vi "PrepareHWI.vi"(8 "error in (no error)":errorcluster, 9 "Master Device in":refnum<class "Master Device.lvclass">, 10 "Current Variables":T1[](array[typedef]), 11 "Slave_Pulseblaster in":refnum<class "Slave_Pulseblaster.lvclass">) -> (0 "error out":errorcluster, 2 "Master Device out":refnum<class "Master Device.lvclass">, 3 "Slave_Pulseblaster out":refnum<class "Slave_Pulseblaster.lvclass">)   [LabVIEW 2013, in "Slave_Pulseblaster.lvclass"]
doc: "Prepare HWI will parse string table values to generate a hardware image for each device. Both variables and user functions can be pre-registered! This makes setting variables optional."
uses:
  Slave_Pulseblaster.lvclass
  TypeDefs/Active procedure variables.ctl
  Master Device/Master Device.lvclass
  Slave_Pulseblaster.lvclass/Slave_Pulseblaster.ctl
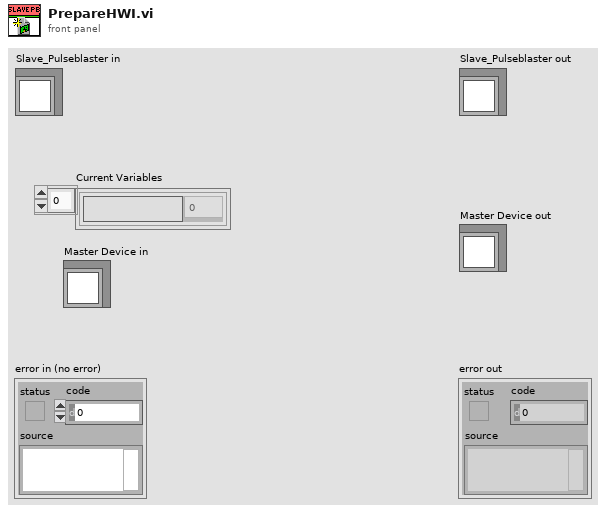
[diagram p1: front panel]
types:
  T1 = typedef "Active procedure variables.ctl" = cluster{"Procedure variable":string, "Value":dbl}
  T2 = cluster{"Output Bits":u32, "Data Field":u32, "OP Code":u8, "Delay Count":u64}[]
  T3 = cluster{"Output Bits":u32, "Data Field":u32, "OP Code":u8, "Delay Count":u64}
  T4 = typedef "SlaveInfo.ctl" = cluster{"Triggering":bool[][], "Ramp Info":T5[], "Line Inversion":bool[]}
  T5 = typedef "RampInfo.ctl" = cluster{"Table Ramp Index":i32, "Ramp Time":dbl, "Number of Steps":i32, "Instruction Array Index":i32}
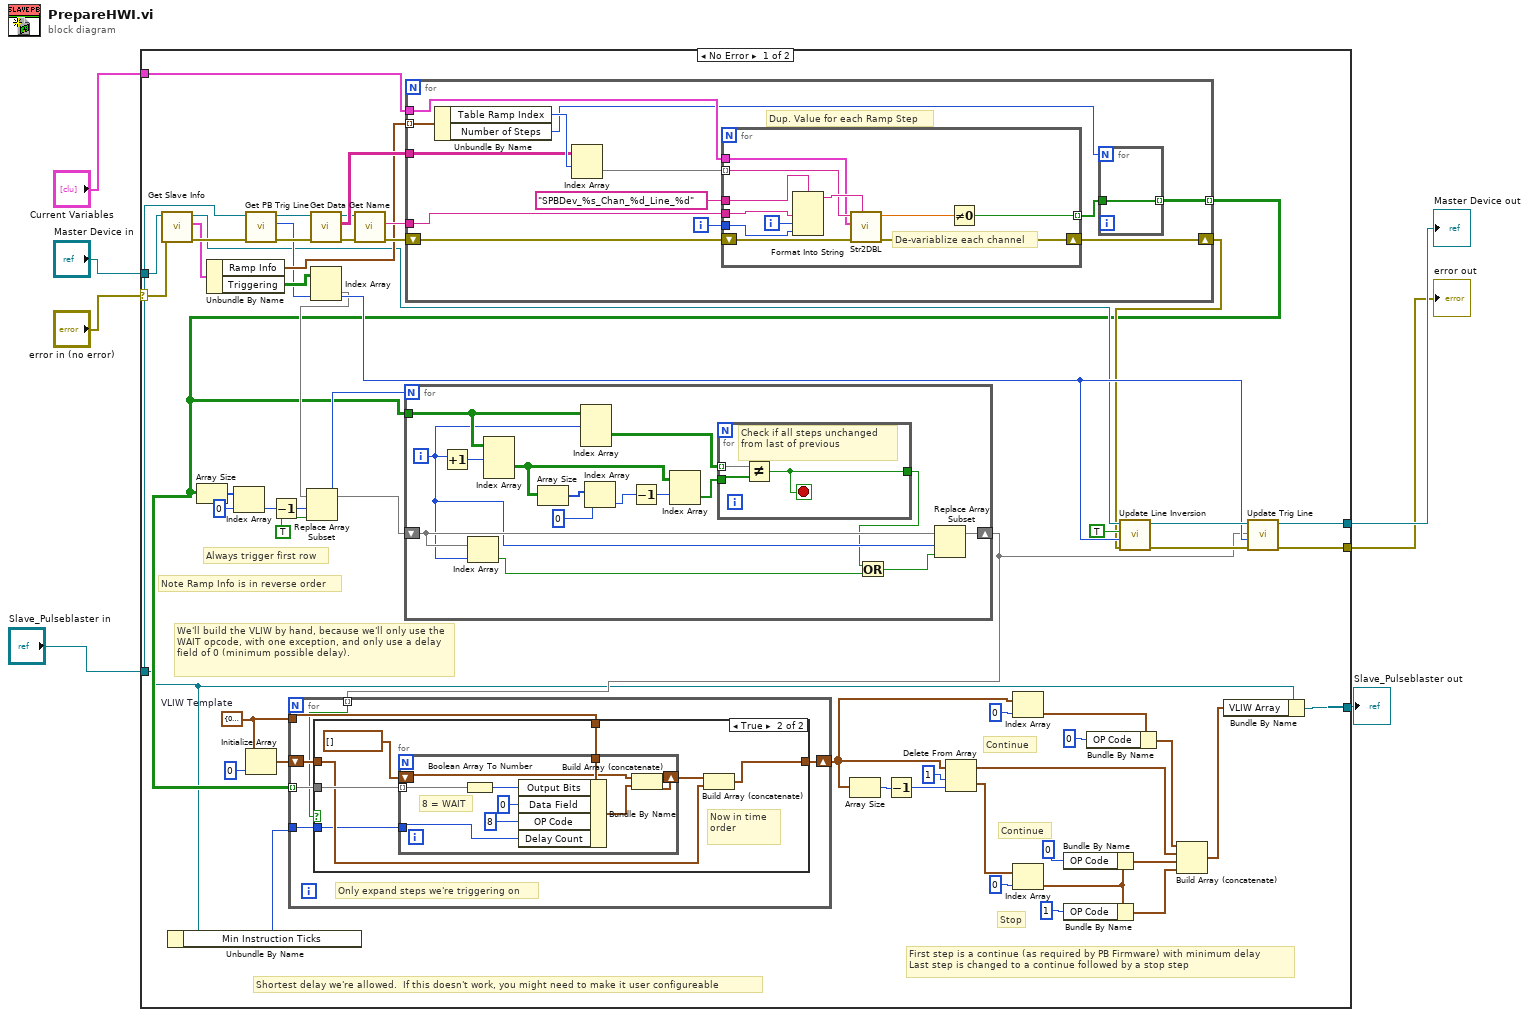
[diagram p0: block diagram]
diagram:
  n1 = case shown="No Error" "error in (no error)" {
    selector: "error in (no error)" -> [w41 w129]
    tunnel: "Master Device in" -> [w50 w130]
    tunnel: "Slave_Pulseblaster in" -> [w9 w128]
    tunnel: "Current Variables" -> [w49 _]
    tunnel: [w47 w130] -> w4
    tunnel: [w44 w129] -> w3
    tunnel: [w27 w128] -> w1
    frame No Error {
      w30 = T3 {"Output Bits"=0, "Data Field"=0, "OP Code"=0, "Delay Count"=0}  # VLIW Template
      # "Shortest delay we're allowed.  If this doesn't work, you might need to make it user configureable"
      # "Continue"
      # "First step is a continue (as required by PB Firmware) with minimum delay\nLast step is changed to a continue followed by a stop step"
      # "Stop"
      # "Continue"
      # "We'll build the VLIW by hand, because we'll only use the WAIT opcode, with one exception, and only use a delay field of 0 (minimum possible delay)."
      # "Note Ramp Info is in reverse order"
      # "Always trigger first row"
      n2 = call-dynamic "Get Slave Info.vi"("error in (no error)"=w41, "Master Device in"=w50) -> ("error out"=w52:errorcluster, "Slave Info"=w51:T4, "Master Device out"=w42:refnum<class "Master Device.lvclass">)  [unwired: 7 in]
      n3 = Unbundle By Name(w9) -> ("Min Instruction Ticks"=w8:u8)
      n4 = Unbundle By Name(w51) -> ("Ramp Info"=w57:T5[], "Triggering"=w61:bool[][])
      n5 = call-dynamic "Get PB Trig Line.vi"("error in (no error)"=w52, "Device in"=w9) -> ("error out"=w53:errorcluster, "PB Trigger Line"=w43:u16, "Device out"=w55:refnum<class "Slave_Pulseblaster.lvclass">)  [unwired: 7 in]
      n6 = Initialize Array(w30, 0 ("dimension size")) -> (w32:T2)
      n7 = call-dynamic "Get Data.vi"("error in (no error)"=w53, "Device in"=w55) -> ("error out"=w54:errorcluster, "Table Indicator"=w58:string[][], "Device out"=w56:refnum<class "Slave_Pulseblaster.lvclass">)  [unwired: 6 in]
      n8 = Index Array(array=w61, index (col)=w43) -> (element=w36:bool[])  [unwired: 1 in]
      n9 = call-dynamic "Get Name.vi"("error in (no error)"=w54, "Device in"=w56) -> ("error out"=w60:errorcluster, "Name"=w59:string)  [unwired: 7 in, 1 out]
      n10 = for {
        tunnel: w57 -> [w115] mode=indexing
        tunnel: w58 -> [w113]
        tunnel: w59 -> [w110]
        tunnel: w49 -> [w108]
        shift-right: [w106] -> w33
        shift-left: w60 -> [w107]
        tunnel: [w103] -> w29 mode=indexing
        i -> [w109]
        # "Dup. Value for each Ramp Step"
        n11 = Unbundle By Name(w115) -> ("Table Ramp Index"=w114:i32, "Number of Steps"=w104:i32)
        n12 = Index Array(array=w113, index (row)=w114) -> (element=w112:string[])  [unwired: 1 in]
        n13 = for {
          tunnel: w112 -> [w118] mode=indexing
          tunnel: "SPBDev_%s_Chan_%d_Line_%d" -> [w127]
          tunnel: w110 -> [w126]
          tunnel: w109 -> [w124]
          tunnel: w108 -> [w117]
          tunnel: [w123] -> w105 mode=indexing
          shift-right: [w120] -> w106
          shift-left: w107 -> [w121]
          i -> [w125]
          # "De-variablize each channel"
          n14 = Format Into String(format string=w127, w126, w125, w124) -> (resulting string=w122:string)  [unwired: 2 in, 1 out]
          n15 = call "Str2DBL.vi"("Error Locator"=w122, "error in (no error)"=w121, "Current Variable settings"=w117, "formula"=w118) -> ("error out"=w120:errorcluster, "y value"=w119:dbl)  [unwired: 4 in]
          n16 = Not Equal To 0?(x=w119) -> (x != 0?=w123:bool)
        }
        n17 = for {
          N: w104 -> [_]
          tunnel: w105 -> [w116]
          tunnel: [w116] -> w103 mode=indexing
        }
      }
      n18 = Array Size(array=w29) -> (size(s)=w37:i32[])
      n19 = Index Array(array=w37, index=0) -> (element=w38:i32)
      n20 = Decrement(x=w38) -> (x-1=w35:i32)
      n21 = Replace Array Subset(array=w36, new element=TRUE ("new element/subarray"), index=w35) -> (w34:bool[])
      n22 = for {
        N: w35 -> [_]
        tunnel: w29 -> [w92]
        shift-right: [w89] -> w28
        shift-left: w34 -> [w90]
        i -> [w88]
        n23 = Increment(x=w88) -> (x+1=w96:i32)
        n24 = Index Array(array=w90, index=w88) -> (element=w87:bool)
        n25 = Index Array(array=w92, index (dim 0)=w96) -> (element=w94:bool[][])  [unwired: 2 in]
        n26 = Array Size(array=w94) -> (size(s)=w99:i32[])
        n27 = Index Array(array=w92, index (dim 0)=w88) -> (element=w91:bool[][])  [unwired: 2 in]
        n28 = Index Array(array=w99, index=0) -> (element=w97:i32)
        n29 = Decrement(x=w97) -> (x-1=w95:i32)
        n30 = Index Array(array=w94, index (row)=w95) -> (element=w93:bool[])  [unwired: 1 in]
        n31 = for {
          tunnel: w93 -> [w102]
          tunnel: [w101] -> w86
          tunnel: w91 -> [w100] mode=indexing
          stop <- w101 stop-if-true
          # "Check if all steps unchanged from last of previous"
          n32 = Not Equal?(x=w100, y=w102) -> (x != y?=w101:bool)
        }
        n33 = Or(x=w86, y=w87) -> (x .or. y?=w85:bool)
        n34 = Replace Array Subset(array=w90, new element=w85, index=w88) -> (w89:bool[])
      }
      n35 = for {
        tunnel: w30 -> [w67]
        shift-right: [w63] -> w24
        shift-left: w32 -> [w66]
        tunnel: w29 -> [w65] mode=indexing
        tunnel: w28 -> [w64] mode=indexing
        tunnel: w8 -> [w62]
        # "Only expand steps we're triggering on"
        n36 = case shown="True" w64 {
          tunnel: w67 -> [_ w75]
          tunnel: w66 -> [w68 w71]
          tunnel: [w68 w72] -> w63
          tunnel: w65 -> [_ w74]
          tunnel: w62 -> [_ w69]
          frame False {
          }
          frame True {
            # "Now in time order"
            n37 = for {
              tunnel: w75 -> [w84]
              shift-right: [w78] -> w73
              shift-left: T2 [] -> [w79]
              tunnel: w74 -> [w77] mode=indexing
              tunnel: w69 -> [w76]
              # "8 = WAIT"
              n38 = Boolean Array To Number(Boolean array=w77) -> (number=w81:u32)
              n39 = Bundle By Name(cluster=w84, "Output Bits"=w81, "Data Field"=u32 0, "OP Code"=u8 8, "Delay Count"=w76) -> (w80:T3)
              n40 = Build Array (concatenate)(w79, w80) -> (w78:T2)
            }
            n41 = Build Array (concatenate)(w73, w71) -> (w72:T2)
          }
        }
      }
      n42 = Array Size(array=w24) -> (size(s)=w25:i32)
      n43 = Decrement(x=w25) -> (x-1=w23:i32)
      n44 = Delete From Array(array=w24, length=1, index=w23) -> (deleted portion=w21:T2, array with subset deleted=w13:T2)
      n45 = Index Array(array=w24, index=0) -> (element=w16:T3)
      n46 = Index Array(array=w21, index=0) -> (element=w19:T3)
      n47 = Bundle By Name(cluster=w19, "OP Code"=u8 0) -> (w12:T3)
      n48 = Bundle By Name(cluster=w19, "OP Code"=u8 1) -> (w11:T3)
      n49 = Bundle By Name(cluster=w16, "OP Code"=u8 0) -> (w14:T3)
      n50 = call-dynamic "Update Line Inversion.vi"("error in (no error)"=w33, "Output Line"=w43, "Invert Line"=TRUE, "Master Device in"=w42) -> ("error out"=w45:errorcluster, "Master Device out"=w48:refnum<class "Master Device.lvclass">)  [unwired: 6 in]
      n51 = Build Array (concatenate)(w14, w13, w12, w11) -> (w10:T2)
      n52 = Bundle By Name(cluster=w9, "VLIW Array"=w10) -> (w27:refnum<class "Slave_Pulseblaster.lvclass">)
      n53 = call-dynamic "Update Trig Line.vi"("error in (no error)"=w45, "Trigger Line"=w43, "Triggering"=w28, "Master Device in"=w48) -> ("error out"=w44:errorcluster, "Master Device out"=w47:refnum<class "Master Device.lvclass">)  [unwired: 6 in]
    }
    frame Error {
    }
  }
  "error out" <- w3
  "Slave_Pulseblaster out" <- w1
  "Master Device out" <- w4
